vi "I2C_0227.vi"() -> ()   [LabVIEW 2021]
doc: "This example demonstrates how to generate a user-defined voltage using the analog output of a DAQ device."
uses:
  <vilib>/Utility/error.llb/DialogType.ctl
  <vilib>/DAQmx/write.llb/DAQmx Write (Digital 1D U32 NChan 1Samp).vi
  <vilib>/DAQmx/create/channels.llb/DAQmx Create Channel (DO-Digital Output).vi
  <vilib>/Utility/file.llb/Read Delimited Spreadsheet (DBL).vi
  <vilib>/DAQmx/miscellaneous.llb/DAQmx Fill In Error Info.vi
panel:
  out "DUT":i32
  out "Numeric":i8
  out "Boolean array":bool[](array[boolean])
  in  "value":bool
  out "DIO":cluster{i16, i16, i16, i16, i16}(graph)
  in  "file path (dialog if empty)":path=path "C:/Users/Wayne Shih/Downloads/nPM6100 Positron/HTOL/Labview/AWG by USB6259/test.txt"
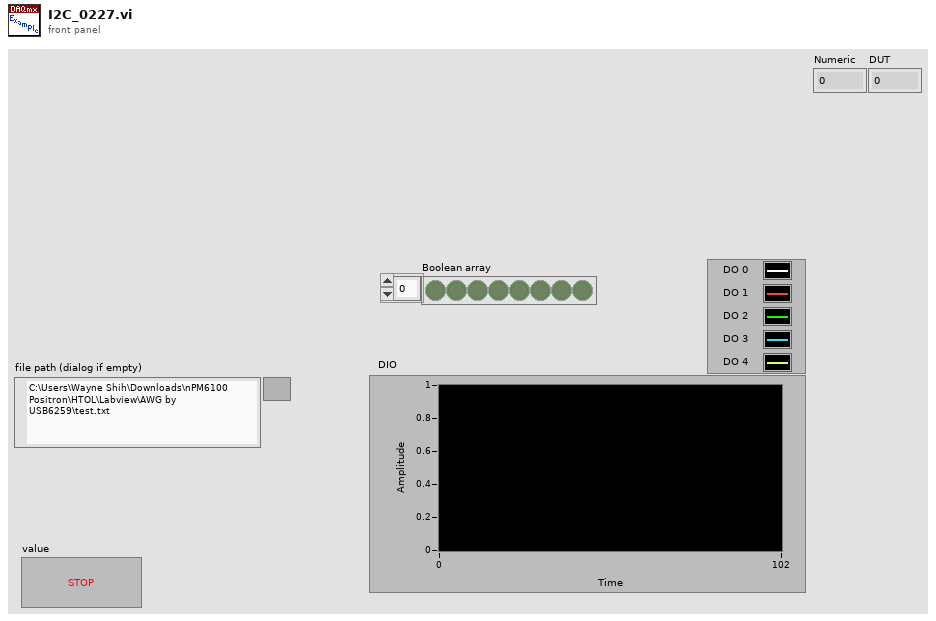
[diagram p1: front panel]
types:
  T1 = typedef "DialogType.ctl" = u16
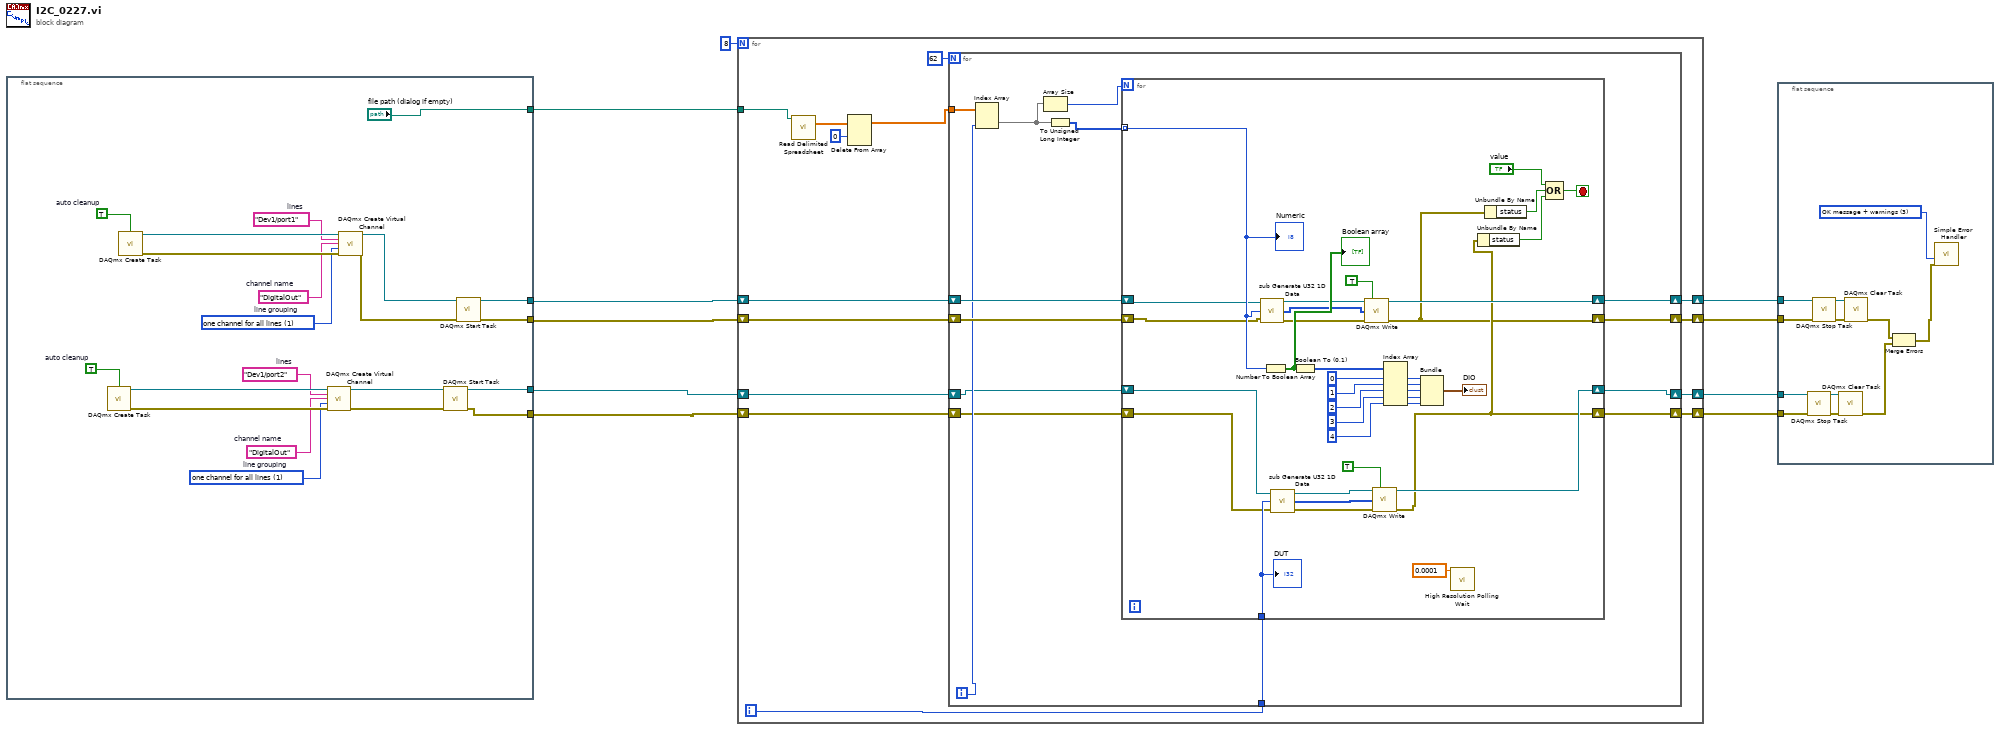
[diagram p0: block diagram]
diagram:
  n1 = flat-sequence {
    tunnel: [w14] -> w10
    tunnel: [w13] -> w9
    tunnel: [w18] -> w5
    tunnel: [w17] -> w4
    tunnel: ["file path (dialog if empty)"] -> w1
    frame #0 {
      w20 = 1 items=["one channel for each line", "one channel for all lines"]  # line grouping
      w19 = "DigitalOut"  # channel name
      w21 = "Dev1/port1"  # lines
      w23 = TRUE  # auto cleanup
      w26 = 1 items=["one channel for each line", "one channel for all lines"]  # line grouping
      w25 = "DigitalOut"  # channel name
      w27 = "Dev1/port2"  # lines
      w29 = TRUE  # auto cleanup
      n2 = call <vilib>:"DAQmx Create Task.vi"("auto cleanup"=w29) -> ("task out"=w28:refnum<k21>, "error out"=w30:errorcluster)  [unwired: 13 in]
      n3 = call <vilib>:"DAQmx Create Task.vi"("auto cleanup"=w23) -> ("task out"=w22:refnum<k21>, "error out"=w24:errorcluster)  [unwired: 13 in]
      n4 = call-poly <vilib>:"DAQmx Create Virtual Channel.vi"("task in"=w28, "lines"=w27, "name to assign"=w25, "line grouping"=w26, "error in"=w30) -> ("task out"=w15:refnum<k21>, "error out"=w16:errorcluster)  [unwired: 9 in]
      n5 = call-poly <vilib>:"DAQmx Create Virtual Channel.vi"("task in"=w22, "lines"=w21, "name to assign"=w19, "line grouping"=w20, "error in"=w24) -> ("task out"=w11:refnum<k21>, "error out"=w12:errorcluster)  [unwired: 9 in]
      n6 = call <vilib>:"DAQmx Start Task.vi"("task/channels in"=w15, "error in"=w16) -> ("task out"=w18:refnum<k21>, "error out"=w17:errorcluster)  [unwired: 12 in]
      n7 = call <vilib>:"DAQmx Start Task.vi"("task/channels in"=w11, "error in"=w12) -> ("task out"=w14:refnum<k21>, "error out"=w13:errorcluster)  [unwired: 12 in]
    }
  }
  n8 = for {
    N: 8 -> [_]
    shift-right: [w43] -> w8
    shift-left: w10 -> [w45]
    shift-right: [w42] -> w7
    shift-left: w9 -> [w44]
    shift-right: [w37] -> w2
    shift-left: w5 -> [w36]
    shift-right: [w38] -> w3
    shift-left: w4 -> [w39]
    tunnel: w1 -> [w33]
    i -> [w40]
    n9 = call-poly <vilib>:"Read Delimited Spreadsheet.vi"("file path (dialog if empty)"=w33) -> ("all rows"=w35:dbl[][])  [unwired: 9 in, 5 out]
    n10 = Delete From Array(array=w35, index (row)=0) -> (array with subset deleted=w32:dbl[][])  [unwired: 2 in, 1 out]
    n11 = for {
      N: 62 -> [_]
      tunnel: w32 -> [w54]
      shift-right: [w57] -> w43
      shift-left: w45 -> [w59]
      shift-right: [w56] -> w42
      shift-left: w44 -> [w58]
      tunnel: w40 -> [w50]
      shift-right: [w47] -> w37
      shift-left: w36 -> [w46]
      shift-right: [w48] -> w38
      shift-left: w39 -> [w49]
      i -> [w51]
      n12 = Index Array(array=w54, index (col)=w51) -> (element=w55:dbl[])  [unwired: 1 in]
      n13 = Array Size(array=w55) -> (size(s)=w53:i32)
      n14 = To Unsigned Long Integer(number=w55) -> (unsigned 32bit integer=w52:u32[])
      n15 = for {
        N: w53 -> [_]
        shift-right: [w95] -> w57
        shift-left: w59 -> [w77]
        shift-right: [w61] -> w56
        shift-left: w58 -> [w76]
        tunnel: w52 -> [w78] mode=indexing
        tunnel: w50 -> [w69]
        shift-right: [w66] -> w47
        shift-left: w46 -> [w68]
        shift-right: [w65] -> w48
        shift-left: w49 -> [w67]
        stop <- w82 stop-if-true
        n16 = call <vilib>:"sub Generate U32 1D Data.vi"("error in"=w76, "initial value"=w78, "task in"=w77) -> ("error out"=w74:errorcluster, "Data"=w75:u32[], "task out"=w73:refnum<k21>)
        n17 = Number To Boolean Array(number=w78) -> (Boolean array=w79:bool[])
        "Boolean array" <- w79
        n18 = call <vilib>:"sub Generate U32 1D Data.vi"("error in"=w67, "initial value"=w69, "task in"=w68) -> ("error out"=w72:errorcluster, "Data"=w71:u32[], "task out"=w70:refnum<k21>)
        n19 = Boolean To (0,1)(Boolean=w79) -> (0, 1=w94:i16[])
        n20 = call-poly <vilib>:"DAQmx Write.vi"("task/channels in"=w73, "auto start"=TRUE, "data"=w75, "error in"=w74) -> ("task out"=w95:refnum<k21>, "error out"=w61:errorcluster)  [unwired: 9 in, 1 out]
        n21 = call-poly <vilib>:"DAQmx Write.vi"("task/channels in"=w70, "auto start"=TRUE, "data"=w71, "error in"=w72) -> ("task out"=w66:refnum<k21>, "error out"=w65:errorcluster)  [unwired: 9 in, 1 out]
        n22 = Index Array(array=w94, index #1=0 ("index"), index #2=1 ("index"), index #3=2 ("index"), index #4=3 ("index"), index #5=4 ("index")) -> (element #1=w88:i16, element #2=w87:i16, element #3=w86:i16, element #4=w85:i16, element #5=w84:i16)
        n23 = Bundle(w88, w87, w86, w85, w84) -> (→"DIO":cluster{i16, i16, i16, i16, i16})  [unwired: 1 in]
        n24 = call <vilib>:"High Resolution Polling Wait.vi"("seconds to wait"=0.0001) -> ()  [unwired: 10 in, 1 out]
        n25 = Unbundle By Name(w65) -> ("status"=w64:bool)
        n26 = Unbundle By Name(w61) -> ("status"=w80:bool)
        n27 = Compound Arithmetic op=OR("value", w80, w64) -> (w82:bool)
        "Numeric" <- w78
        "DUT" <- w69
      }
    }
  }
  n28 = flat-sequence {
    tunnel: w8 -> [w104]
    tunnel: w7 -> [w103]
    tunnel: w3 -> [w100]
    tunnel: w2 -> [w99]
    frame #0 {
      w107 = T1 3 items=["no dialog", "OK message", "continue or stop message", "OK message + warnings", "continue/stop + warnings"] ("type of dialog (OK msg:1)")
      n29 = call <vilib>:"DAQmx Stop Task.vi"("task/channels in"=w99, "error in"=w100) -> ("task out"=w101:refnum<k21>, "error out"=w102:errorcluster)  [unwired: 12 in]
      n30 = call <vilib>:"DAQmx Stop Task.vi"("task/channels in"=w104, "error in"=w103) -> ("task out"=w105:refnum<k21>, "error out"=w106:errorcluster)  [unwired: 12 in]
      n31 = call <vilib>:"DAQmx Clear Task.vi"("task in"=w101, "error in"=w102) -> ("error out"=w98:errorcluster)  [unwired: 13 in]
      n32 = call <vilib>:"DAQmx Clear Task.vi"("task in"=w105, "error in"=w106) -> ("error out"=w97:errorcluster)  [unwired: 13 in]
      n33 = Merge Errors(w97, w98) -> (w96:errorcluster)
      n34 = call <vilib>:"Simple Error Handler.vi"("type of dialog (OK msg:1)"=w107, "error in (no error)"=w96) -> ()  [unwired: 3 in, 5 out]
    }
  }
